vi "IIR Filter Design - DFD.vi"() -> ()   [LabVIEW 2023]
doc: "Demonstrates how to design an IIR filter using VIs in the LabVIEW Digital Filter Design Toolkit.\n\nYou can select five IIR filter design methods, including Bessel, Butterworth, Chebyshev I and II, and Elliptic, and any passband type, including lowpass, highpass, bandpass, and bandstop."
uses:
  <vilib>/addons/Digital Filter Design/_Objects.llb/DFD Phase Setting.ctl
  <vilib>/addons/Digital Filter Design/Analysis.llb/DFD Plot Freq Response (Linear-Spaced).vi
  <vilib>/addons/Digital Filter Design/NI_DigFilterLicensed.lvlib
panel:
  in  "stop":bool
  out "?":string="dB"
  in  "sampling rate":dbl=1000.0 format="%0.2f"
  in  "Display":bool=TRUE
  in  "Attenuation":dbl=40.0 format="%0.2f"
  in  "Ripple":dbl=10.0 format="%0.2f"
  in  "Higher":dbl=300.0 format="%0.2f"
  in  "Lower":dbl=100.0 format="%0.2f"
  in  "Filter Design":T1(ring)=enum."Elliptic"
  in  "Filter Type":i32(ring)=2 items=["Lowpass", "Highpass", "Bandpass", "Bandstop"]
  in  "Order":i32=4
  out "Phase Response":cluster{"f0":dbl, "df":dbl, "values":dbl[]}[](graph)
  out "Magnitude Response":cluster{"f0":dbl, "df":dbl, "values":dbl[]}[](graph)
  # "Select Help»Show Context Help and move the cursor over the VI icon for more information."
  # "Hz"
  # "radians"
  # "Cut-Off Frequencies"
  # "Hz"
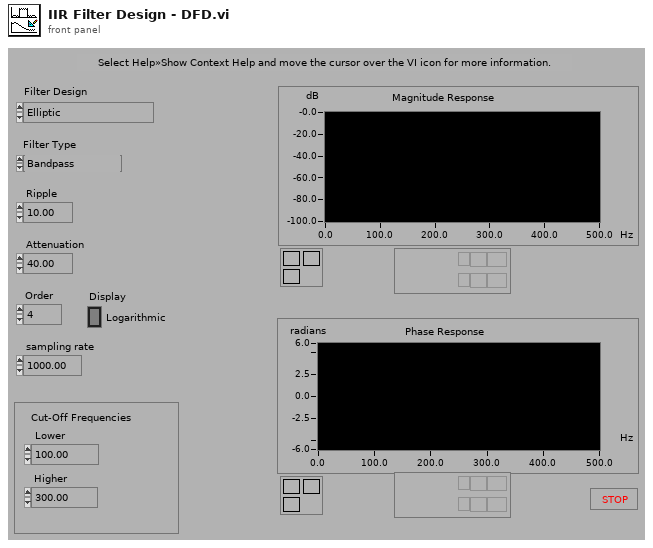
[diagram p1: front panel]
types:
  T1 = enum16{"Butterworth", "Chebyshev", "Inv Chebyshev", "Elliptic", "Bessel"}
  T2 = typedef "NI_DigFilterLicensed.lvlib/DFD Phase Setting.ctl" = cluster{"unwrap? (F)":bool, "degree? (F)":bool}
  T3 = typedef "NI_DigFilterLicensed.lvlib/DFD Filter Obj.ctl" = cluster{"mSRate_Fs":dbl, "mSRate_Version":string, "mSRate_Comments":string, "mSRate_OrgCoef":T4, "mSRate_CurCoef":T4, "mSRate_Quantized?":bool, "mSRate_QCoef":T4, "mSRate_QSettings":T6[], "mSRate_Order":i32, "mSRate_Scaling":cluster{"mSRate_ScaleByPowerOf2?":bool, "mSRate_ScaleType":T8}}
  T4 = typedef "NI_DigFilterLicensed.lvlib/DFD Filter Coef.ctl" = cluster{"type":T5, "gain":dbl, "coef a (k)":dbl[], "coef b (v)":dbl[]}
  T5 = typedef "NI_DigFilterLicensed.lvlib/DFD Filter Structure Type Selector.ctl" = enum16{"Undefined", "FIR Direct Form", "FIR Direct Form Transposed", "FIR Symmetric", "FIR Antisymmetric", "IIR Direct Form I", "IIR Direct Form I Transposed", "IIR Direct Form II", "IIR Direct Form II Transposed", "IIR Cascaded Second Order Sections Form I", "IIR Cascaded Second Order Sections Form I Transposed", "IIR Cascaded Second Order Sections Form II", "IIR Cascaded Second Order Sections Form II Transposed", "Lattice Allpass (basic sections)", "Lattice Allpass (one multiplier sections)", "Lattice Allpass (normalized sections)", "Lattice AR (basic sections)", "Lattice AR (one multiplier sections)", "Lattice AR (normalized sections)", "Lattice MA (minimum phase)", "Lattice MA (maximum phase)", "Lattice ARMA (basic sections)", "Lattice ARMA (one multiplier sections)", "Lattice ARMA (normalized sections)"}
  T6 = typedef "NI_DigFilterLicensed.lvlib/dfd_Internal Quantization Settings.ctl" = cluster{"source":T7, "wl":i16, "iwl":i16, "overflow mode":enum16{"Saturation", "Wrap"}, "rounding mode":enum16{"Nearest", "Truncation"}, "signed?":bool}
  T7 = typedef "NI_DigFilterLicensed.lvlib/dfd_Internal Quantization Srcs.ctl" = u16
  T8 = typedef "NI_DigFilterLicensed.lvlib/DFD Coef Norm Type.ctl" = enum16{"No Norm", "Time Domain 1-Norm", "Time Domain 2-Norm", "Time Domain Inf-Norm"}
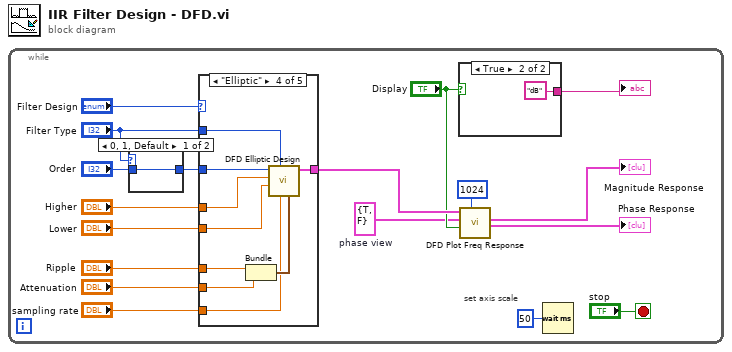
[diagram p0: block diagram]
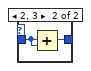
[diagram p2: hidden frame]
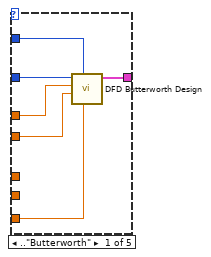
[diagram p3: hidden frame]
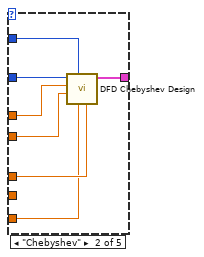
[diagram p4: hidden frame]
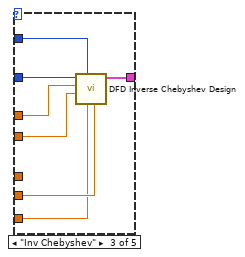
[diagram p5: hidden frame]
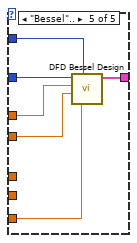
[diagram p6: hidden frame]
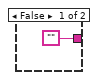
[diagram p7: hidden frame]
diagram:
  n1 = while {
    stop <- "stop" stop-if-true
    w7 = T2 {"unwrap? (F)"=TRUE, "degree? (F)"=FALSE}  # phase view
    # "set axis scale"
    n2 = case shown="0, 1, Default" "Filter Type" {
      tunnel: "Order" -> [w19 w20]
      tunnel: [w19 w21] -> w1
      frame 0, 1, Default {
      }
      frame 2, 3 {
        n3 = Add(x=w20, y=w20) -> (x+y=w21:i32)
      }
    }
    n4 = case shown="\"Elliptic\"" "Filter Design" {
      tunnel: "Filter Type" -> [w24 w34 w41 w48 w56]
      tunnel: "Higher" -> [w27 w33 w40 w50 w55]
      tunnel: "Lower" -> [w26 w32 w39 w49 w54]
      tunnel: w1 -> [w25 w31 w38 w47 w53]
      tunnel: "Ripple" -> [_ w30 _ w46 _]
      tunnel: "Attenuation" -> [_ _ w37 w42 _]
      tunnel: "sampling rate" -> [w23 w29 w36 w43 w52]
      tunnel: [w22 w28 w35 w44 w51] -> w9
      frame .."Butterworth" {
        n5 = call <vilib>:"DFD Butterworth Design.vi"("fs [Hz]"=w23, "filter type"=w24, "low cutoff freq [Hz]"=w26, "high cutoff freq [Hz]"=w27, "order"=w25) -> ("filter out"=w22:T3)  [unwired: 1 in, 5 out]
      }
      frame "Chebyshev" {
        n6 = call <vilib>:"DFD Chebyshev Design.vi"("passband ripple [dB]"=w30, "fs [Hz]"=w29, "filter type"=w34, "low cutoff freq [Hz]"=w32, "high cutoff freq [Hz]"=w33, "order"=w31) -> ("filter out"=w28:T3)  [unwired: 1 in, 4 out]
      }
      frame "Inv Chebyshev" {
        n7 = call <vilib>:"DFD Inverse Chebyshev Design.vi"("stopband atten [dB]"=w37, "fs [Hz]"=w36, "filter type"=w41, "low cutoff freq [Hz]"=w39, "high cutoff freq [Hz]"=w40, "order"=w38) -> ("filter out"=w35:T3)  [unwired: 1 in, 4 out]
      }
      frame "Elliptic" {
        n8 = Bundle("Ripple"=w46, "Attenuation"=w42) -> (w45:cluster{"Ripple":dbl, "Attenuation":dbl})  [unwired: 1 out]
        n9 = call <vilib>:"DFD Elliptic Design.vi"("ripples [dB]"=w45, "fs [Hz]"=w43, "filter type"=w48, "low cutoff freq [Hz]"=w49, "high cutoff freq [Hz]"=w50, "order"=w47) -> ("filter out"=w44:T3)  [unwired: 2 in, 3 out]
      }
      frame "Bessel".. {
        n10 = call <vilib>:"DFD Bessel Design.vi"("fs [Hz]"=w52, "filter type"=w56, "low cutoff freq [Hz]"=w54, "high cutoff freq [Hz]"=w55, "order"=w53) -> ("filter out"=w51:T3)  [unwired: 1 in, 5 out]
      }
    }
    n11 = case shown="True" "Display" {
      tunnel: ["" "dB"] -> w18
      frame False {
      }
      frame True {
      }
    }
    "?" <- w18
    n12 = call-poly <vilib>:"DFD Plot Freq Response.vi"("# freq bins"=1024 ("# freq bins (auto)"), "dB on? (T)"="Display", "phase view"=w7, "filter in"=w9) -> ("phase response"=→"Phase Response":cluster{"f0":dbl, "df":dbl, "values":dbl[]}[], "magnitude response"=→"Magnitude Response":cluster{"f0":dbl, "df":dbl, "values":dbl[]}[])  [unwired: 4 in, 2 out]
    n13 = Wait (ms)(milliseconds to wait=u32 50) -> ()  [unwired: 1 out]
  }
